vi "FisherPaykel Find VISA Resource.vi"(8 "Error In":errorcluster) -> (0 "Error Out":errorcluster, 2 "General Resource Found":bool, 3 "VISA Resource":refnum<visa-resource-name>[](array[refnum]))   [LabVIEW 2016]
uses:
  <vilib>/Instr/_visa.llb/VISA Open Access Mode.ctl
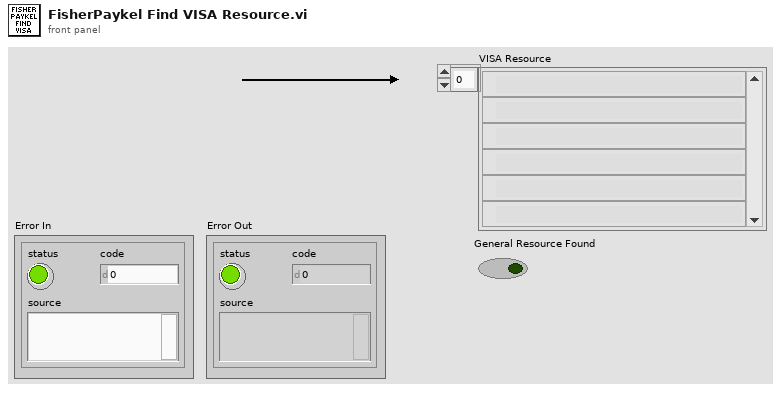
[diagram p1: front panel]
types:
  T1 = typedef "VISA Open Access Mode.ctl" = u32
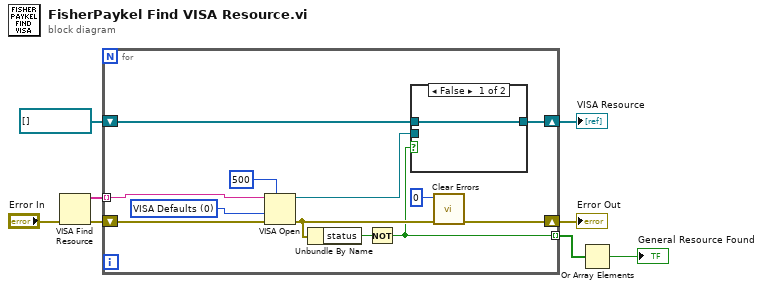
[diagram p0: block diagram]
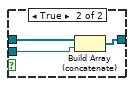
[diagram p2: hidden frame]
diagram:
  n1 = VISA Find Resource(8:"Error In") -> (0:w7:errorcluster, 3:w6:string[])  [unwired: 2 in, 1 out]
  n2 = for {
    tunnel: w6 -> [w20] mode=indexing
    shift-right: [w15] -> w3
    shift-left: w7 -> [w18]
    tunnel: [w12] -> w8 mode=indexing
    shift-right: [w10] -> w2
    shift-left: refnum<visa-resource-name>[] [] -> [w9]
    w19 = T1 0 items=["VISA Defaults"=0, "Exclusive Lock"=1, "Load Configured Settings"=4] ("Access Mode")
    n3 = VISA Open(timeout (0)=u32 500 ("VISA Open timeout (0)"), access mode=w19, error in (no error)=w18, VISA resource name=w20) -> (VISA resource name=w11:refnum<visa-resource-name>, error out=w14:errorcluster)  [unwired: 1 in]
    n4 = Unbundle By Name(w14) -> ("status"=w13:bool)
    n5 = Not(x=w13) -> (.not. x?=w12:bool)
    n6 = case shown="False" w12 {
      tunnel: w11 -> [_ w23]
      tunnel: [w21 w22] -> w10
      tunnel: w9 -> [w21 w24]
      frame False {
      }
      frame True {
        n7 = Build Array (concatenate)(w24, w23) -> (w22:refnum<visa-resource-name>[])
      }
    }
    n8 = call <vilib>:"Clear Errors.vi"("error in (no error)"=w14, "specific error code to clear (0: all)"=0) -> ("error out"=w15:errorcluster)  [unwired: 4 in, 1 out]
  }
  "Error Out" <- w3
  "VISA Resource" <- w2
  n9 = Or Array Elements(Boolean array=w8) -> (logical OR=→"General Resource Found":bool)
